vi "Read side.vi"(8 "error in (no error)":errorcluster, 11 "Room":refnum<class "Room.lvclass">) -> (0 "error out":errorcluster, 2 "sides":refnum<class "MazeSite.lvclass">[](array[class]), 3 "Room":refnum<class "Room.lvclass">)   [LabVIEW 2020, in "Room.lvclass"]
uses:
  Room.lvclass
  MazeSite/MazeSite.lvclass
  Room.lvclass/Room.ctl
  TypeDef/privateDataDVR.ctl
  TypeDef/privateData.ctl
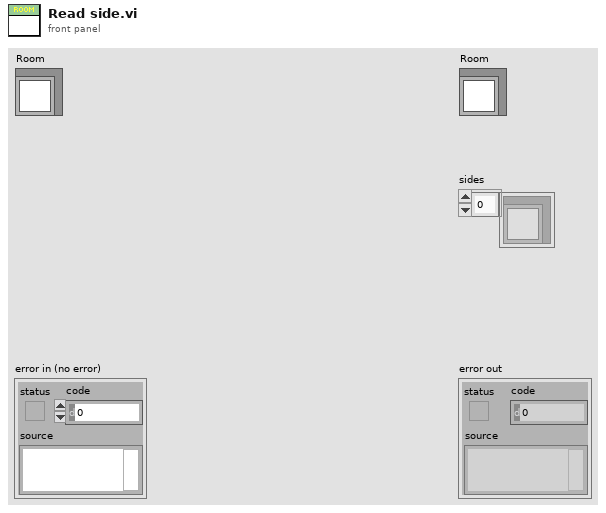
[diagram p1: front panel]
types:
  T1 = typedef "Room.lvclass/privateDataDVR.ctl" = refnum<data-value>
  T2 = typedef "Room.lvclass/privateData.ctl" = cluster{"sides":refnum<class "MazeSite.lvclass">[], "roomNumber":i32}
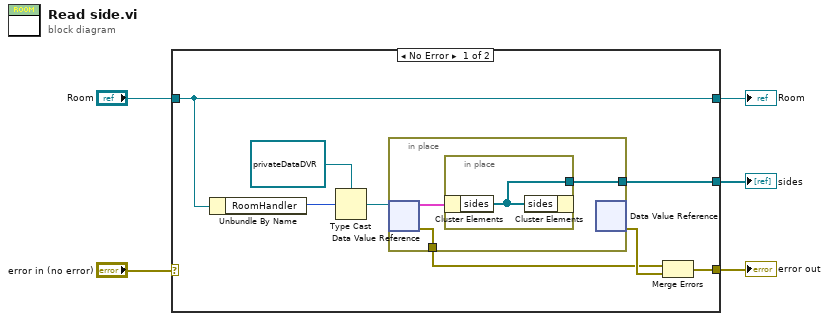
[diagram p0: block diagram]
diagram:
  n1 = case shown="No Error" "error in (no error)" {
    selector: "error in (no error)" -> [_ w18]
    tunnel: "Room" -> [w9 w19]
    tunnel: [w9 w19] -> w4
    tunnel: [w8 w18] -> w3
    tunnel: [w6 _] -> w1
    frame No Error {
      n2 = Unbundle By Name(w9) -> ("RoomHandler"=w11:u32)
      n3 = Type Cast(type=T1 refnum ("privateDataDVR"), x=w11) -> (*(type *) &x=w13:T1)
      n4 = in-place {
        in-place-border: [w15] -> w10
        in-place-border: [w14] -> w6
        n5 = in-place-dvr #1(w13) -> (w16:T2, w15:errorcluster)
        n6 = in-place {
          in-place-border: [w17] -> w14
          n7 = in-place-cluster #2(w16) -> ("sides"=w17:refnum<class "MazeSite.lvclass">[])
          n8 = in-place-cluster #2("sides"=w17) -> ()  [unwired: 1 out]
        }
        n9 = in-place-dvr #1() -> (w12:errorcluster)  [unwired: 1 in, 1 out]
      }
      n10 = Merge Errors(w10, w12) -> (w8:errorcluster)
    }
    frame Error {
    }
  }
  "error out" <- w3
  "Room" <- w4
  "sides" <- w1
